vi "Grab Hatch Panel in Auto (BEDPC-GB8-7's conflicted copy 2019-03-16).vi"   [LabVIEW 2018]
uses:
  SubSystems/Hatch Panel Intake/Hatch Panel Intake Global.vi
  SubSystems/Cargo Intake/Cargo Intake Global.vi
  SubSystems/Lift/Lift Global.vi
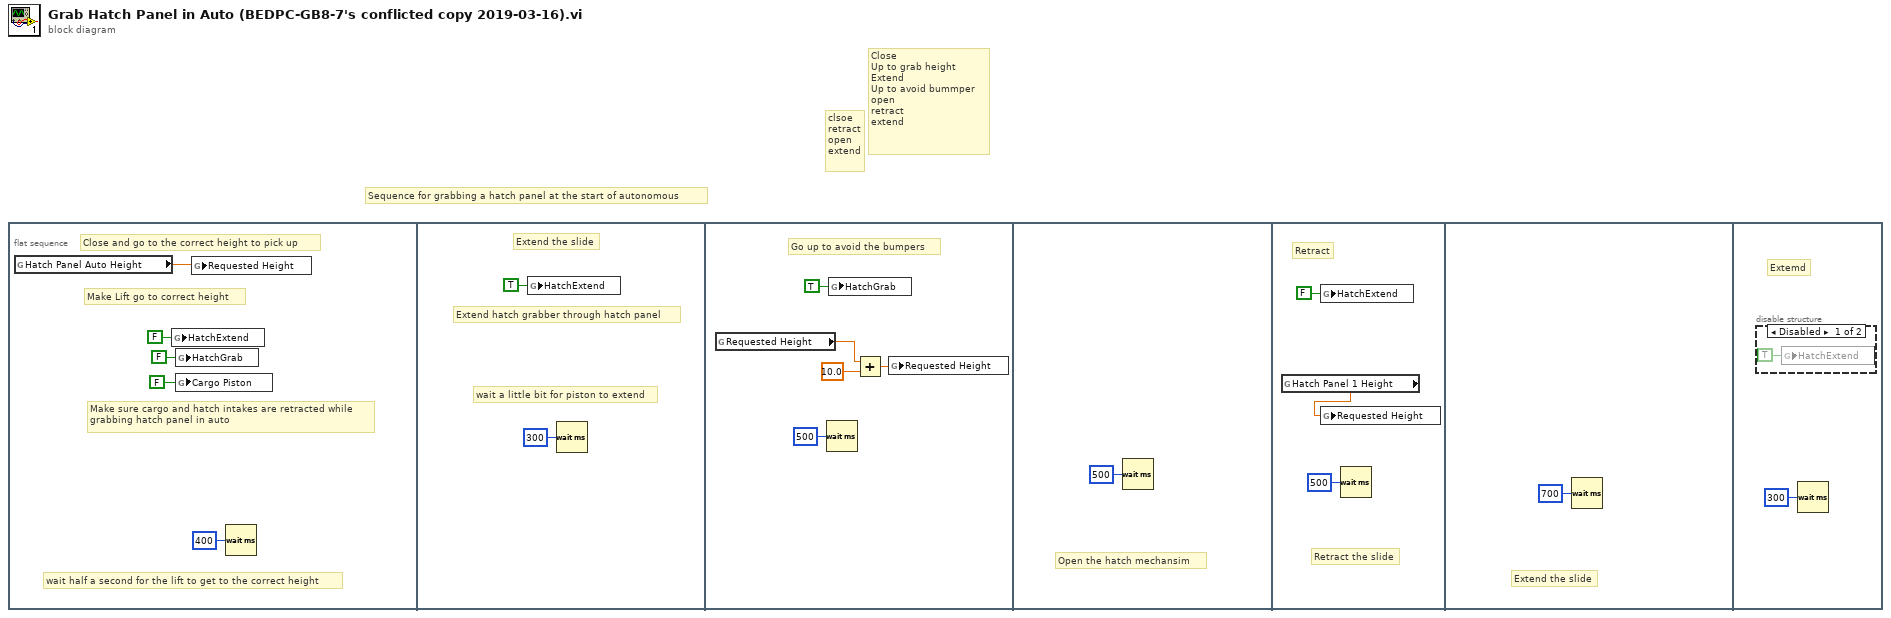
[diagram p0: block diagram]
diagram:
  # "clsoe\nretract\nopen\nextend"
  # "Close\nUp to grab height\nExtend\nUp to avoid bummper\nopen\nretract\nextend"
  # "Sequence for grabbing a hatch panel at the start of autonomous"
  n1 = flat-sequence {
    frame #0 {
      # "Close and go to the correct height to pick up"
      # "Make sure cargo and hatch intakes are retracted while\ngrabbing hatch panel in auto"
      # "wait half a second for the lift to get to the correct height"
      # "Make Lift go to correct height"
      n2 = global read "Lift Global.vi" "Hatch Panel Auto Height"() -> (w5:dbl)
      n3 = global write "Hatch Panel Intake Global.vi" "HatchExtend"(FALSE ("HatchExtend")) -> ()
      n4 = global write "Hatch Panel Intake Global.vi" "HatchGrab"(FALSE ("HatchGrab")) -> ()
      n5 = global write "Cargo Intake Global.vi" "Cargo Piston"(FALSE ("Cargo Piston")) -> ()
      n6 = global write "Lift Global.vi" "Requested Height"(w5) -> ()
      n7 = Wait (ms)(milliseconds to wait=u32 400) -> ()  [unwired: 1 out]
    }
    frame #1 {
      # "Extend the slide"
      # "wait a little bit for piston to extend"
      # "Extend hatch grabber through hatch panel"
      n8 = global write "Hatch Panel Intake Global.vi" "HatchExtend"(TRUE ("HatchExtend")) -> ()
      n9 = Wait (ms)(milliseconds to wait=u32 300) -> ()  [unwired: 1 out]
    }
    frame #2 {
      # "Go up to avoid the bumpers"
      n10 = global read "Lift Global.vi" "Requested Height"() -> (w10:dbl)
      n11 = Wait (ms)(milliseconds to wait=u32 500) -> ()  [unwired: 1 out]
      n12 = global write "Hatch Panel Intake Global.vi" "HatchGrab"(TRUE ("HatchGrab")) -> ()
      n13 = Add(x=w10, y=10.0) -> (x+y=w11:dbl)
      n14 = global write "Lift Global.vi" "Requested Height"(w11) -> ()
    }
    frame #3 {
      # "Open the hatch mechansim"
      n15 = Wait (ms)(milliseconds to wait=u32 500) -> ()  [unwired: 1 out]
    }
    frame #4 {
      # "Retract"
      # "Retract the slide"
      n16 = global read "Lift Global.vi" "Hatch Panel 1 Height"() -> (w14:dbl)
      n17 = global write "Hatch Panel Intake Global.vi" "HatchExtend"(FALSE ("HatchExtend")) -> ()
      n18 = global write "Lift Global.vi" "Requested Height"(w14) -> ()
      n19 = Wait (ms)(milliseconds to wait=u32 500) -> ()  [unwired: 1 out]
    }
    frame #5 {
      # "Extend the slide"
      n20 = Wait (ms)(milliseconds to wait=u32 700) -> ()  [unwired: 1 out]
    }
    frame #6 {
      # "Extemd"
      n21 = disable-structure shown="Disabled" {
        frame Disabled {
          n22 = global write "Hatch Panel Intake Global.vi" "HatchExtend"(TRUE ("HatchExtend")) -> ()
        }
        frame Enabled {
        }
      }
      n23 = Wait (ms)(milliseconds to wait=u32 300) -> ()  [unwired: 1 out]
    }
  }
